vi "Autonomous Independent.vi"   [LabVIEW 2016]
doc: "This VI is called when autonomous begins, and will automatically be terminated when autonomous ends. You can carry out timed or sensor driven robot movement independently without needing to return to the caller."
uses:
  <vilib>/Rock Robotics/WPI/Ultrasonic/WPI_UltrasonicRangeUnits.ctl
  <vilib>/Rock Robotics/WPI/ThirdParty/Sensors/navX/_TypeDefs/FRIC_navX_DeviceNumbersTypeDef.ctl
  <vilib>/Rock Robotics/WPI/Utilities/WPI_GetSetVariantRefNum.vi
  <vilib>/Rock Robotics/Network Tables/NT Read String.vi
  <vilib>/Rock Robotics/Network Tables/NT Write Numeric Array.vi
  Robot Global Data.vi
  <vilib>/Rock Robotics/WPI/RobotDrive/WPI_RobotDriveArcadeDrive_Standard(NoSaturation).vi
  <vilib>/Rock Robotics/WPI/Ultrasonic/WPI_SonarSRF04DigitalRefNum Registry Get.vi
  <vilib>/Rock Robotics/WPI/Ultrasonic/WPI_SonarSRF04DigitalGetRange.vi
panel:
  # "Be sure to right-click and choose Data Operations>>Make Current Value default if you want to save the array values with the VI"
types:
  T1 = typedef "WPI_JoystickDevRef.ctl" = cluster{"Device":T2}
  T2 = typedef "WPI_JoystickDeviceEnum.ctl" = enum16{"USB 0", "USB 1", "USB 2", "USB 3", "USB 4", "USB 5"}
  T3 = typedef "WPI_UltrasonicRangeUnits.ctl" = enum16{"inches", "mm"}
  T4 = typedef "WPI_RobotDriveDevRef.ctl" = cluster{"DevStatus":errorcluster, "Motors[]":T5[], "Square Inputs":bool, "Max Output":dbl}
  T5 = typedef "WPI_MotorControlDeviceRef.ctl" = cluster{"DeviceStatus":errorcluster, "Type":T6, "PWM":cluster{"PWM Channel":T7, "DeadBand":T8}, "CAN":cluster{"Device Number":u8, "SetOutput VI Ref":variant, "GetOutput VI Ref":variant, "Enable VI Ref":variant, "Disable VI Ref":variant, "Data":variant}, "Invert":bool}
  T6 = typedef "WPI_MotorControlType.ctl" = enum16{"PWM", "CAN"}
  T7 = typedef "FPGA_DIOPWMChannel.ctl" = enum8{"PWM 0", "PWM 1", "PWM 2", "PWM 3", "PWM 4", "PWM 5", "PWM 6", "PWM 7", "PWM 8", "PWM 9", "PWM MXP 0", "PWM MXP 1", "PWM MXP 2", "PWM MXP 3", "PWM MXP 4", "PWM MXP 5", "PWM MXP 6", "PWM MXP 7", "PWM MXP 8", "PWM MXP 9", "Invalid"}
  T8 = typedef "WPI_PWMDeadband.ctl" = cluster{"Name":string, "maxPositivePwm":i32, "minPositivePwm":i32, "centerPwm":i32, "maxNegativePwm":i32, "minNegativePwm":i32, "angularRange":u16}
  T9 = cluster{"Type":enum16{"Normal Object", "Color Object"}, "Signature":u16, "X":u16, "Y":u16, "Width":u16, "Height":u16, "Angle":u16}[]
  T10 = cluster{"Type":enum16{"Normal Object", "Color Object"}, "Signature":u16, "X":u16, "Y":u16, "Width":u16, "Height":u16, "Angle":u16}
  T11 = typedef "WPI_UltrasonicDeviceRef.ctl" = cluster{"DevStatus":errorcluster, "Ping Channel":T12, "Echo Channel":T12, "CntIndex":T13}
  T12 = typedef "FPGA_DIOChannel.ctl" = enum8{"DIO 0", "DIO 1", "DIO 2", "DIO 3", "DIO 4", "DIO 5", "DIO 6", "DIO 7", "DIO 8", "DIO 9", "DIO MXP 0", "DIO MXP 1", "DIO MXP 2", "DIO MXP 3", "DIO MXP 4", "DIO MXP 5", "DIO MXP 6", "DIO MXP 7", "DIO MXP 8", "DIO MXP 9", "DIO MXP 10", "DIO MXP 11", "DIO MXP 12", "DIO MXP 13", "DIO MXP 14", "DIO MXP 15", "SPI Port CS1", "SPI Port CS2", "SPI Port CS3", "SPI Port MISO", "SPI Port MOSI", "Invalid"}
  T13 = typedef "FPGA_CounterCtrSystemIndex.ctl" = enum8{"Ctr 0", "Ctr 1", "Ctr 2", "Ctr 3", "Ctr 4", "Ctr 5", "Ctr 6", "Ctr 7", "Invalid"}
  T14 = typedef "FRIC_navX_DeviceNumbersTypeDef.ctl" = enum16{"Dev0", "Dev1", "Dev2", "Dev3"}
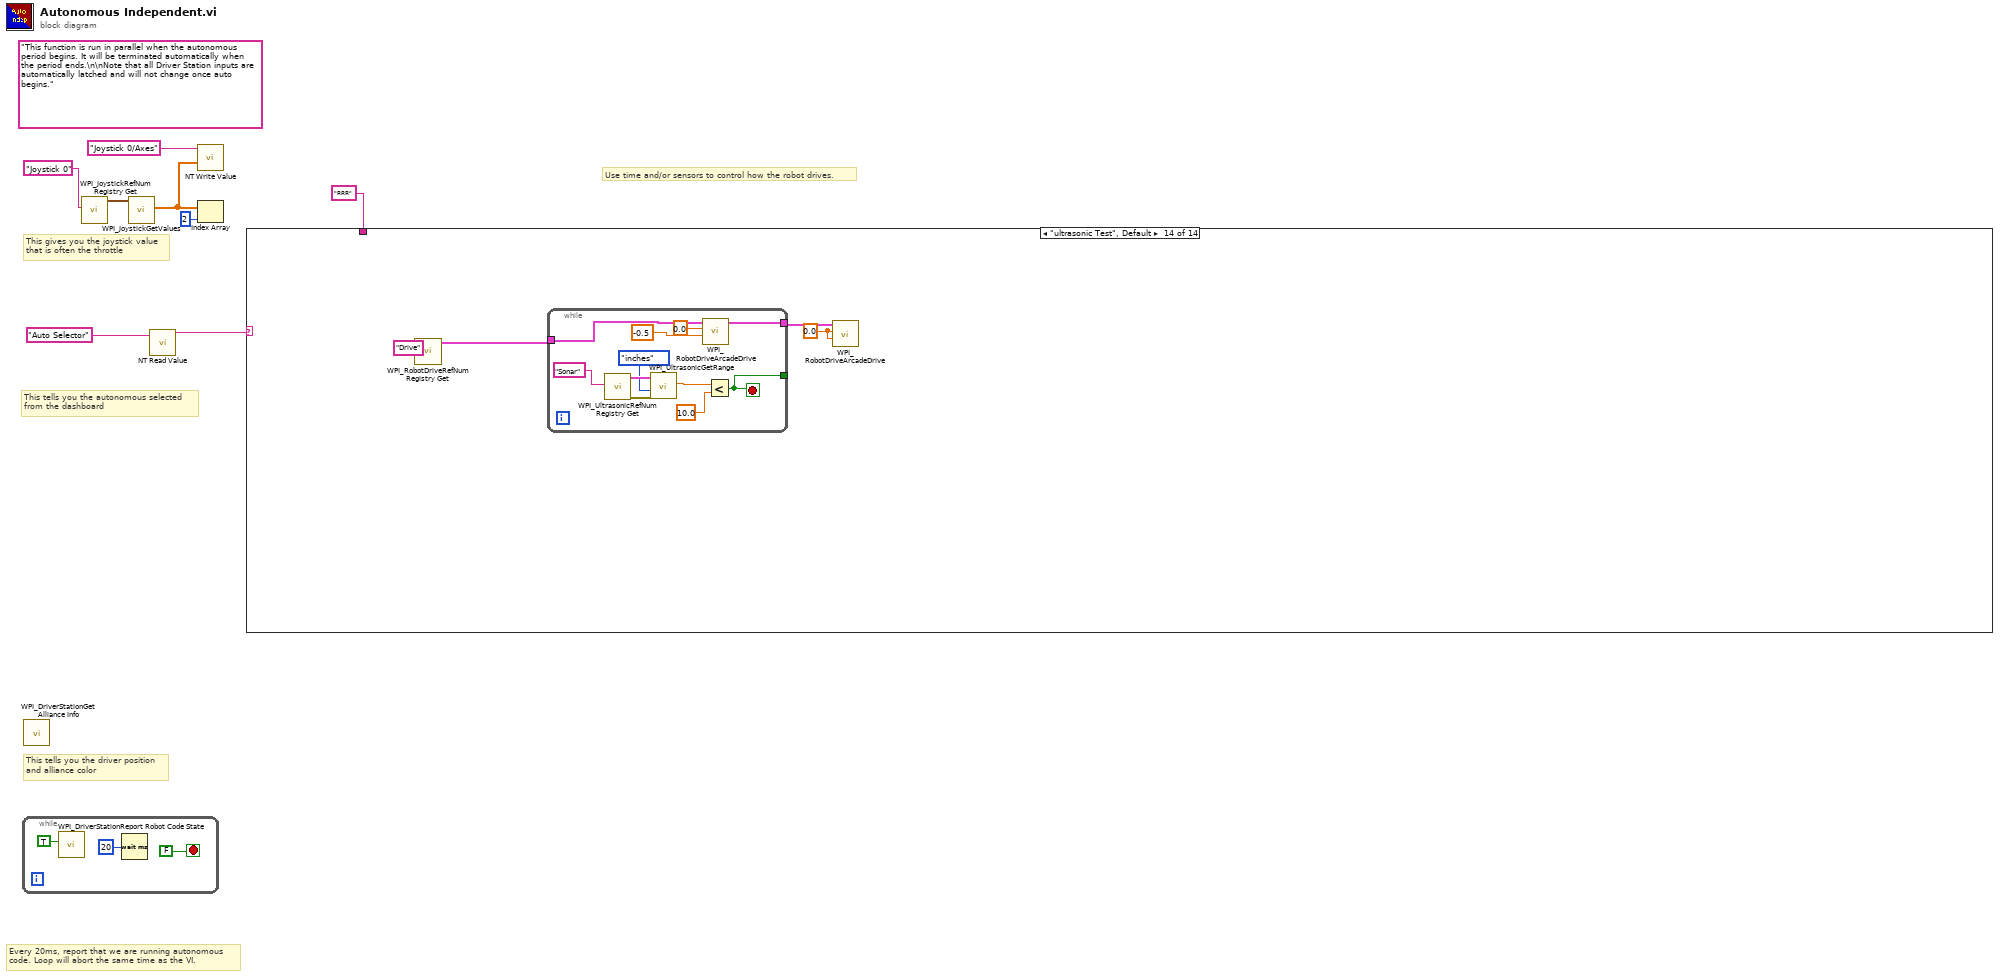
[diagram p0: block diagram]
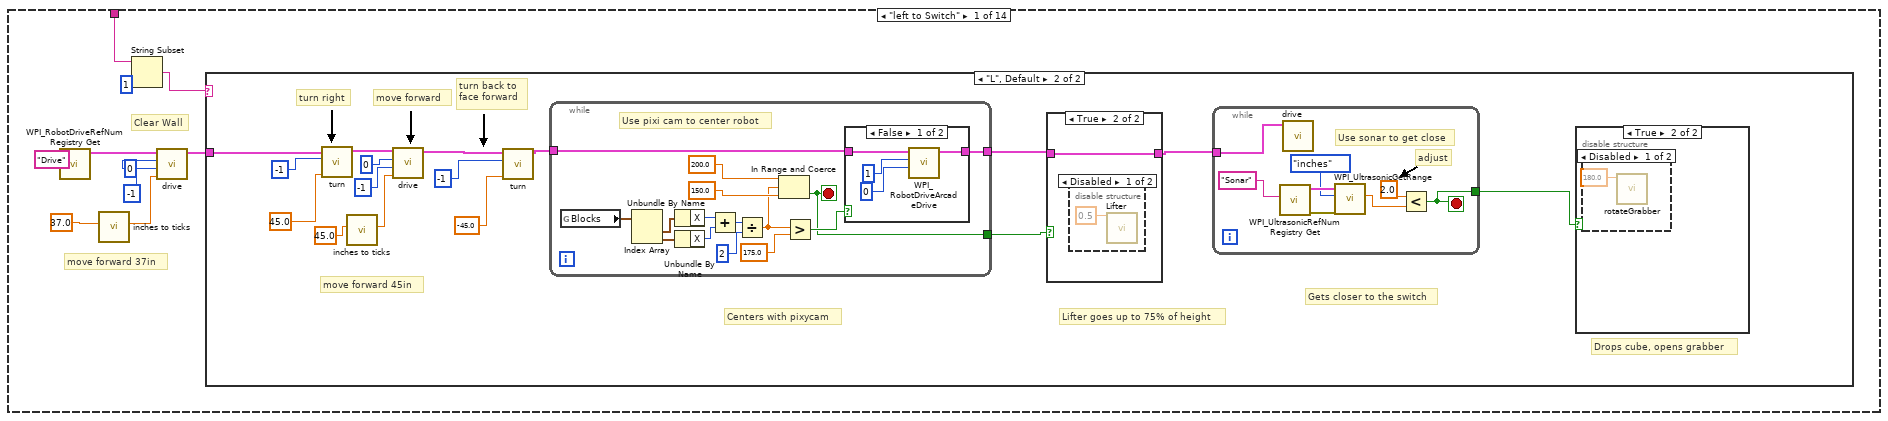
[diagram p2: hidden frame]
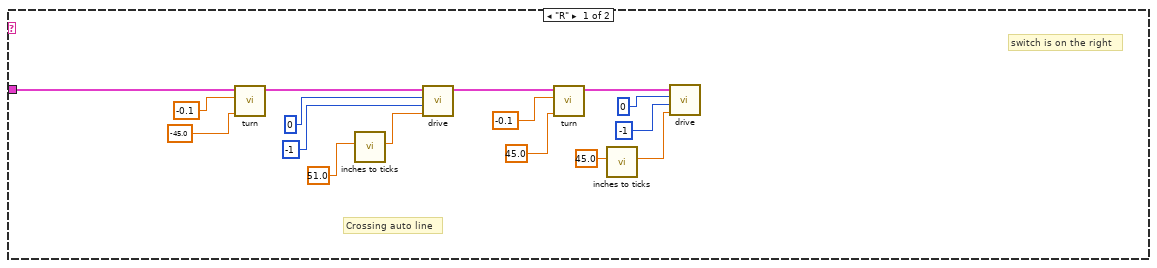
[diagram p3: hidden frame]
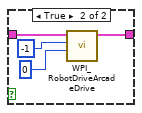
[diagram p8: hidden frame]
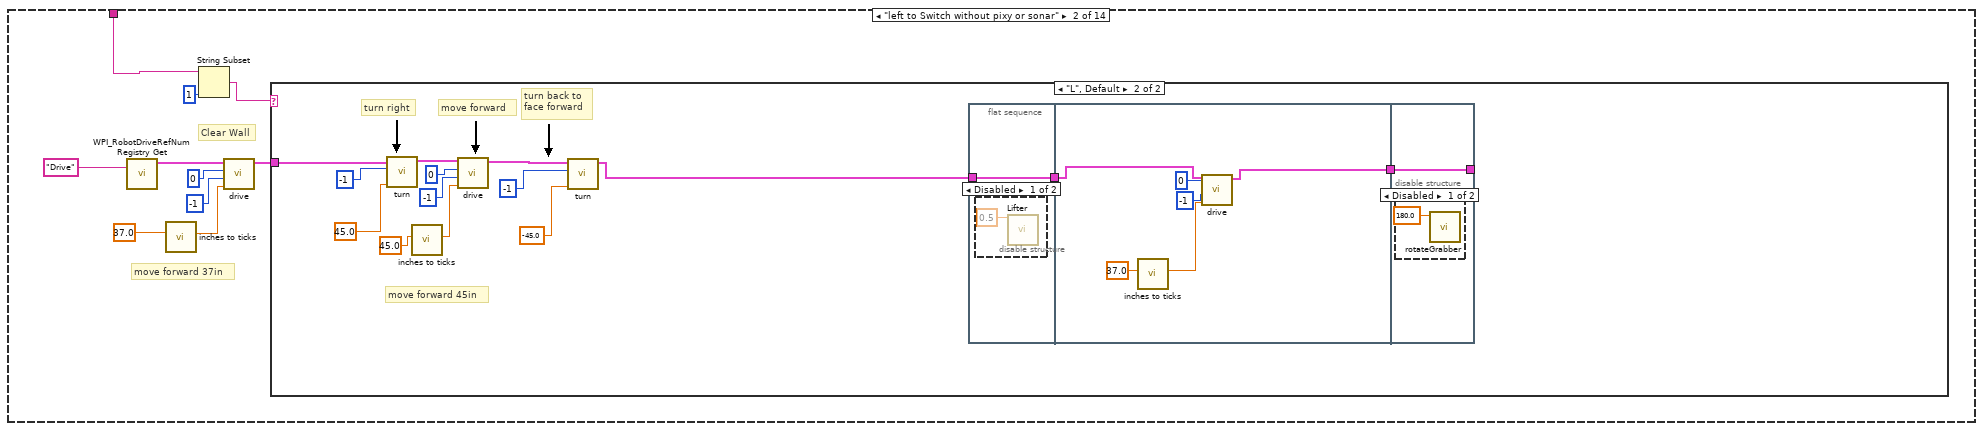
[diagram p9: hidden frame]
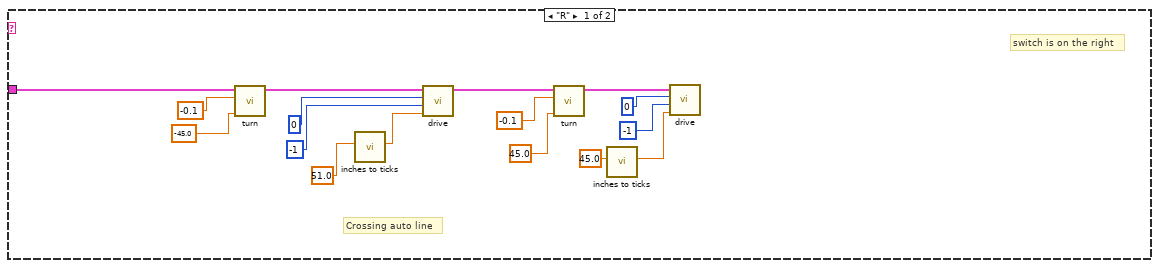
[diagram p10: hidden frame]
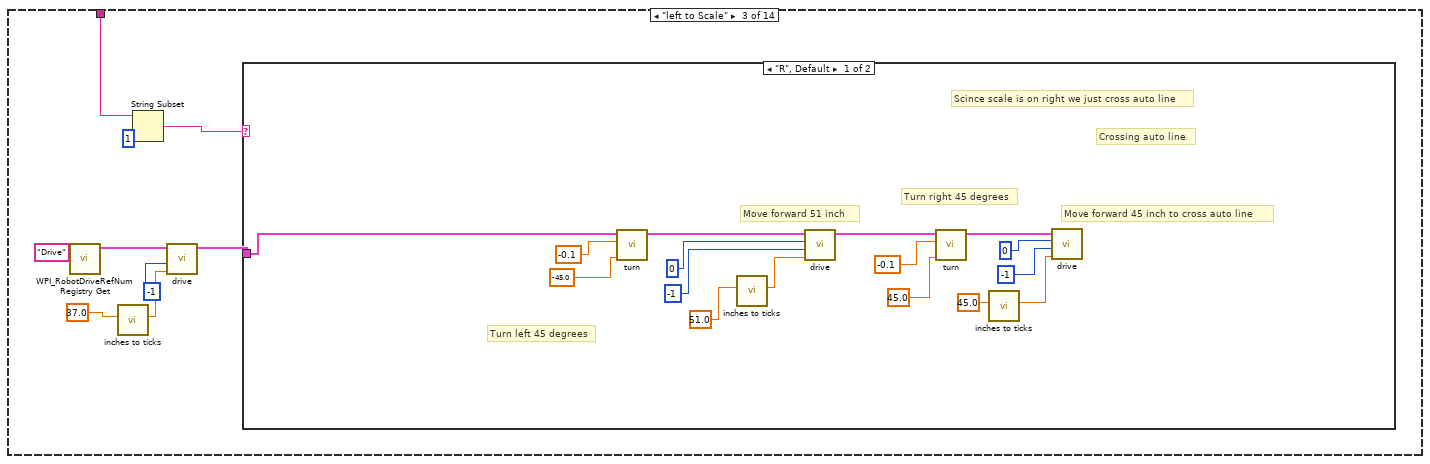
[diagram p13: hidden frame]
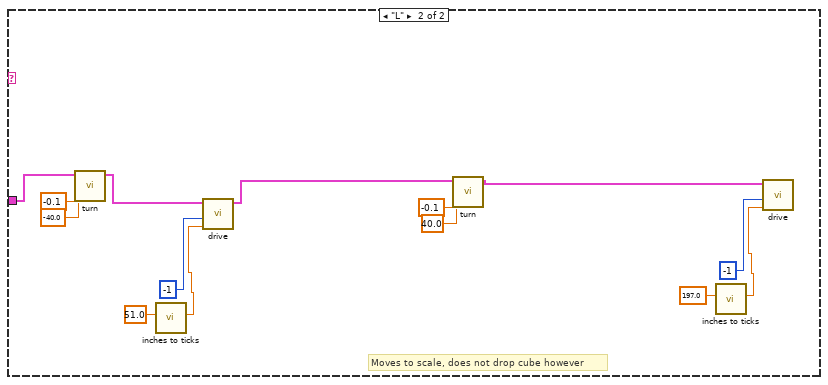
[diagram p14: hidden frame]
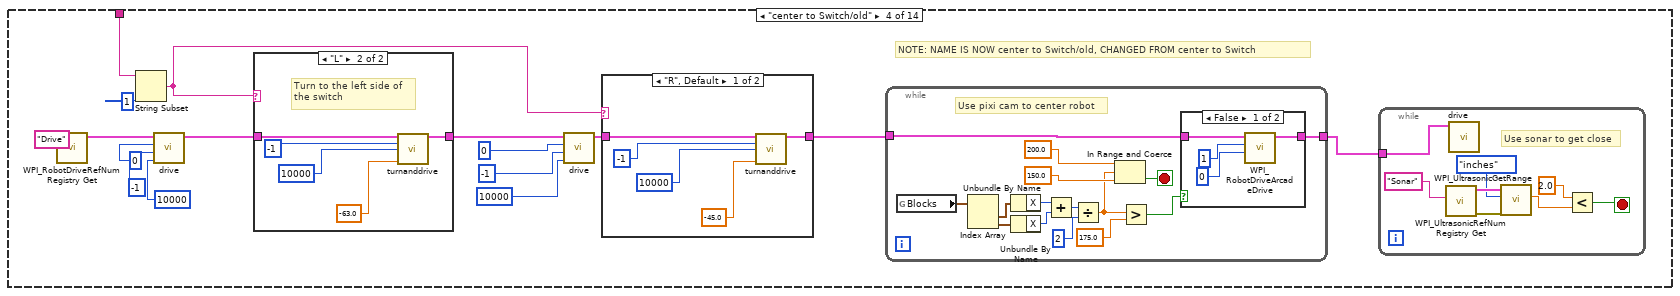
[diagram p15: hidden frame]
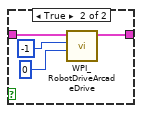
[diagram p16: hidden frame]
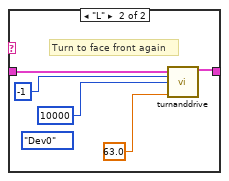
[diagram p17: hidden frame]
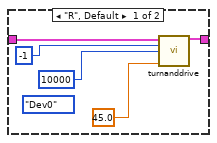
[diagram p18: hidden frame]
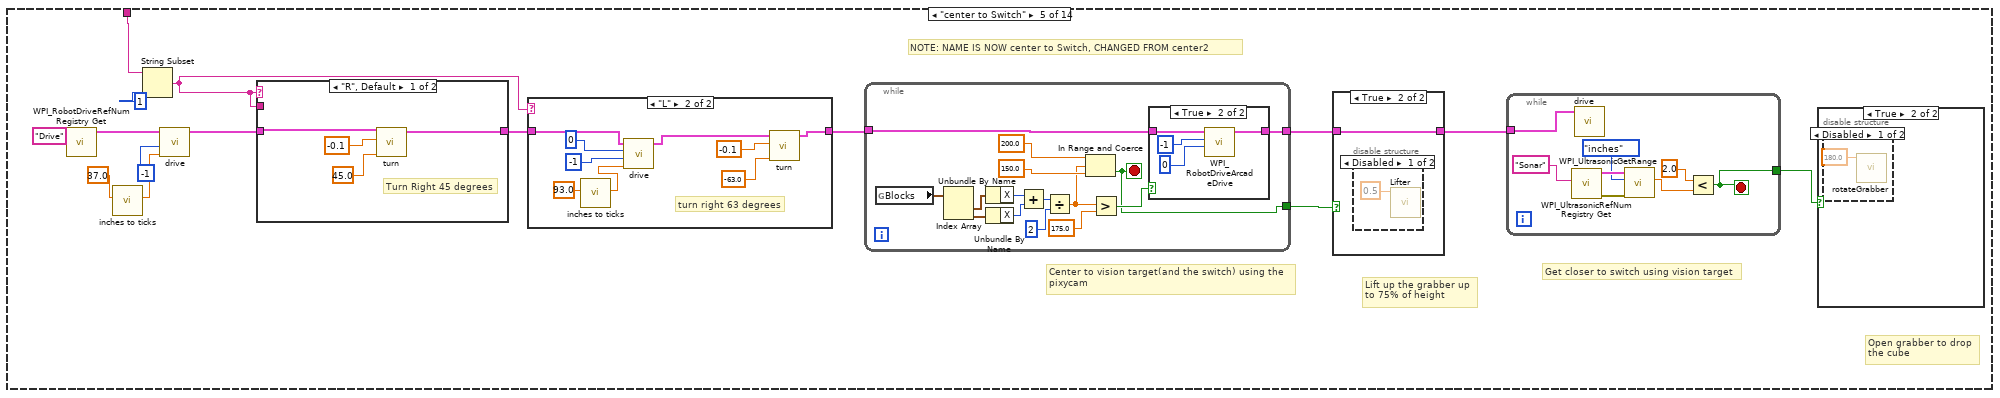
[diagram p19: hidden frame]
diagram:
  (unwired) "This function is run in parallel when the autonomous period begins. It will be terminated automatically when the period ends.\n\nNote that all Driver Station inputs are automatically latched and will not change once auto begins."
  # "This tells you the autonomous selected\nfrom the dashboard"
  # "Every 20ms, report that we are running autonomous\ncode. Loop will abort the same time as the VI."
  # "This gives you the joystick value\nthat is often the throttle"
  # "Use time and/or sensors to control how the robot drives."
  # "This tells you the driver position\nand alliance color"
  n1 = while {
    stop <- FALSE stop-if-true
    n2 = call <vilib>:"WPI_DriverStationReport Robot Code State.vi"("Autonomous"=TRUE) -> ()  [unwired: 10 in, 1 out]
    n3 = Wait (ms)(milliseconds to wait=u32 20) -> ()  [unwired: 1 out]
  }
  n4 = call <vilib>:"WPI_DriverStationGet Alliance Info.vi"() -> ()  [unwired: 12 out]
  n5 = call <vilib>:"WPI_JoystickRefNum Registry Get.vi"("refnum name"="Joystick 0") -> ("JoystickDevRef"=w7:T1)  [unwired: 1 in, 9 out]
  n6 = call <vilib>:"WPI_JoystickGetValues.vi"("JoystickDevRef"=w7) -> ("Axes"=w4:dbl[])  [unwired: 6 in, 4 out]
  n7 = call-poly <vilib>:"NT Read Value.vi"("Name"="Auto Selector") -> ("String"=w2:string)  [unwired: 9 in, 1 out]
  n8 = call-poly <vilib>:"NT Write Value.vi"("Numeric Array"=w4, "Name"="Joystick 0/Axes") -> ()  [unwired: 9 in, 1 out]
  n9 = Index Array(array=w4, index=2) -> ()  [unwired: 1 out]
  n10 = case shown="\"ultrasonic Test\", Default" w2 {
    tunnel: "RRR" ("String") -> [w12 w89 w139 w178 w245 w321 _ _ _ w402 w479 w530 w575 _]
    frame "left to Switch" {
      # "move forward 37in"
      # "Clear Wall"
      n11 = call <vilib>:"WPI_RobotDriveRefNum Registry Get.vi"("refnum name"="Drive") -> ("RobotDriveDevRef"=w20:T4)  [unwired: 9 in, 1 out]
      n12 = call "inches to ticks.vi"("x"=37.0) -> ("x*y"=w14:dbl)  [unwired: 10 in]
      n13 = String Subset(string=w12, length (rest)=1 ("length (rest)")) -> (substring=w15:string)  [unwired: 1 in]
      n14 = call "drive.vi"("distance"=w14, "Y"=-1, "X"=0, "RobotDriveDevRef"=w20) -> ("RobotDriveDevRef dup."=w16:T4)  [unwired: 7 in]
      n15 = case shown="\"L\", Default" w15 {
        tunnel: w16 -> [w22 w53]
        frame "R" {
          # "Crossing auto line"
          # "switch is on the right"
          n16 = call "turn.vi"("Angle"=-45.0, "y"=-0.1, "RobotDriveDevRef"=w22) -> ("RobotDriveDevRef dup."=w31:T4)  [unwired: 8 in]
          n17 = call "inches to ticks.vi"("x"=51.0) -> ("x*y"=w37:dbl)  [unwired: 10 in]
          n18 = call "drive.vi"("distance"=w37, "Y"=-1, "X"=0, "RobotDriveDevRef"=w31) -> ("RobotDriveDevRef dup."=w29:T4)  [unwired: 7 in]
          n19 = call "turn.vi"("Angle"=45.0, "y"=-0.1, "RobotDriveDevRef"=w29) -> ("RobotDriveDevRef dup."=w27:T4)  [unwired: 8 in]
          n20 = call "inches to ticks.vi"("x"=45.0) -> ("x*y"=w26:dbl)  [unwired: 10 in]
          n21 = call "drive.vi"("distance"=w26, "Y"=-1, "X"=0, "RobotDriveDevRef"=w27) -> ()  [unwired: 7 in, 1 out]
        }
        frame "L", Default {
          # "Drops cube, opens grabber"
          # "Gets closer to the switch"
          # "Lifter goes up to 75% of height"
          # "Centers with pixycam"
          # "move forward 45in"
          # "turn back to \nface forward"
          # "move forward"
          # "turn right"
          n22 = call "turn.vi"("Angle"=45.0, "y"=-1, "RobotDriveDevRef"=w53) -> ("RobotDriveDevRef dup."=w50:T4)  [unwired: 8 in]
          n23 = call "inches to ticks.vi"("x"=45.0) -> ("x*y"=w43:dbl)  [unwired: 10 in]
          n24 = call "drive.vi"("distance"=w43, "Y"=-1, "X"=0, "RobotDriveDevRef"=w50) -> ("RobotDriveDevRef dup."=w48:T4)  [unwired: 7 in]
          n25 = call "turn.vi"("Angle"=-45.0, "y"=-1, "RobotDriveDevRef"=w48) -> ("RobotDriveDevRef dup."=w45:T4)  [unwired: 8 in]
          n26 = while {
            tunnel: w45 -> [w67]
            tunnel: [w68] -> w41
            tunnel: [w66] -> w39
            stop <- w66 stop-if-true
            # "Use pixi cam to center robot"
            n27 = global read "Robot Global Data.vi" "Blocks"() -> (w80:T9)
            n28 = Index Array(array=w80) -> (element #1=w79:T10, element #2=w78:T10)  [unwired: 2 in]
            n29 = Unbundle By Name(w79) -> ("X"=w77:u16)
            n30 = Unbundle By Name(w78) -> ("X"=w76:u16)
            n31 = Add(x=w77, y=w76) -> (x+y=w75:u16)
            n32 = Divide(x=w75, y=u16 2) -> (x/y=w73:dbl)
            n33 = In Range and Coerce(upper limit=200.0, x=w73, lower limit=150.0) -> (In Range?=w66:bool)  [unwired: 1 out]
            n34 = Greater?(x=w73, y=175.0) -> (0:w71:bool)
            n35 = case shown="False" w71 {
              tunnel: w67 -> [w84 w86]
              tunnel: [w81 w85] -> w68
              frame False {
                n36 = call-poly <vilib>:"WPI_RobotDriveArcadeDrive.vi"("Y axis value"=0, "X axis value"=1, "RobotDriveDevRef"=w84) -> ("RobotDriveDevRef"=w81:T4)  [unwired: 6 in, 2 out]
              }
              frame True {
                n37 = call-poly <vilib>:"WPI_RobotDriveArcadeDrive.vi"("Y axis value"=0, "X axis value"=-1, "RobotDriveDevRef"=w86) -> ("RobotDriveDevRef"=w85:T4)  [unwired: 6 in, 2 out]
              }
            }
          }
          n38 = case shown="True" w39 {
            tunnel: [w55 w56] -> w40
            tunnel: w41 -> [w55 w56]
            frame False {
            }
            frame True {
              n39 = disable-structure shown="Disabled" {
                frame Disabled {
                  n40 = call "Lifter.vi"("Position from -1 to 1"=0.5) -> ()  [unwired: 11 in]
                }
                frame Enabled {
                }
              }
            }
          }
          n41 = while {
            tunnel: w40 -> [w65]
            tunnel: [w58] -> w38
            stop <- w58 stop-if-true
            # "adjust"
            # "Use sonar to get close"
            n42 = call-poly <vilib>:"WPI_UltrasonicRefNum Registry Get.vi"("refnum name"="Sonar") -> ("error out"=w63:errorcluster, "SonarSRF04DevRef"=w64:T11)  [unwired: 9 in]
            n43 = call "drive.vi"("RobotDriveDevRef"=w65) -> ()  [unwired: 10 in, 1 out]
            n44 = call-poly <vilib>:"WPI_UltrasonicGetRange.vi"("error in (no error)"=w63, "ping time (s)"=WPI_UltrasonicRangeUnits."inches" ("Range Units"), "SonarSRF04DevRef"=w64) -> ("Distance"=w61:dbl)  [unwired: 6 in, 2 out]
            n45 = Less?(x=2.0, y=w61) -> (x < y?=w58:bool)
          }
          n46 = case shown="True" w38 {
            frame False {
            }
            frame True {
              n47 = disable-structure shown="Disabled" {
                frame Disabled {
                  n48 = call "rotateGrabber.vi"("Position from 90 to 180"=180.0) -> ()  [unwired: 11 in]
                }
                frame Enabled {
                }
              }
            }
          }
        }
      }
    }
    frame "left to Switch without pixy or sonar" {
      # "move forward 37in"
      # "Clear Wall"
      n49 = call <vilib>:"WPI_RobotDriveRefNum Registry Get.vi"("refnum name"="Drive") -> ("RobotDriveDevRef"=w95:T4)  [unwired: 9 in, 1 out]
      n50 = call "inches to ticks.vi"("x"=37.0) -> ("x*y"=w98:dbl)  [unwired: 10 in]
      n51 = String Subset(string=w89, length (rest)=1 ("length (rest)")) -> (substring=w97:string)  [unwired: 1 in]
      n52 = call "drive.vi"("distance"=w98, "Y"=-1, "X"=0, "RobotDriveDevRef"=w95) -> ("RobotDriveDevRef dup."=w96:T4)  [unwired: 7 in]
      n53 = case shown="\"L\", Default" w97 {
        tunnel: w96 -> [w99 w128]
        frame "R" {
          # "Crossing auto line"
          # "switch is on the right"
          n54 = call "turn.vi"("Angle"=-45.0, "y"=-0.1, "RobotDriveDevRef"=w99) -> ("RobotDriveDevRef dup."=w108:T4)  [unwired: 8 in]
          n55 = call "inches to ticks.vi"("x"=51.0) -> ("x*y"=w114:dbl)  [unwired: 10 in]
          n56 = call "drive.vi"("distance"=w114, "Y"=-1, "X"=0, "RobotDriveDevRef"=w108) -> ("RobotDriveDevRef dup."=w106:T4)  [unwired: 7 in]
          n57 = call "turn.vi"("Angle"=45.0, "y"=-0.1, "RobotDriveDevRef"=w106) -> ("RobotDriveDevRef dup."=w104:T4)  [unwired: 8 in]
          n58 = call "inches to ticks.vi"("x"=45.0) -> ("x*y"=w103:dbl)  [unwired: 10 in]
          n59 = call "drive.vi"("distance"=w103, "Y"=-1, "X"=0, "RobotDriveDevRef"=w104) -> ()  [unwired: 7 in, 1 out]
        }
        frame "L", Default {
          # "move forward 45in"
          # "turn back to \nface forward"
          # "move forward"
          # "turn right"
          n60 = call "turn.vi"("Angle"=45.0, "y"=-1, "RobotDriveDevRef"=w128) -> ("RobotDriveDevRef dup."=w125:T4)  [unwired: 8 in]
          n61 = call "inches to ticks.vi"("x"=45.0) -> ("x*y"=w119:dbl)  [unwired: 10 in]
          n62 = call "drive.vi"("distance"=w119, "Y"=-1, "X"=0, "RobotDriveDevRef"=w125) -> ("RobotDriveDevRef dup."=w123:T4)  [unwired: 7 in]
          n63 = call "turn.vi"("Angle"=-45.0, "y"=-1, "RobotDriveDevRef"=w123) -> ("RobotDriveDevRef dup."=w116:T4)  [unwired: 8 in]
          n64 = flat-sequence {
            tunnel: [w129] -> w117
            tunnel: w116 -> [w129]
            tunnel: w117 -> [w132]
            tunnel: [w131] -> w115
            tunnel: w115 -> [w137]
            tunnel: [w137] -> _
            frame #0 {
              n65 = disable-structure shown="Disabled" {
                frame Disabled {
                  n66 = call "Lifter.vi"("Position from -1 to 1"=0.5) -> ()  [unwired: 11 in]
                }
                frame Enabled {
                }
              }
            }
            frame #1 {
              n67 = call "inches to ticks.vi"("x"=37.0) -> ("x*y"=w136:dbl)  [unwired: 10 in]
              n68 = call "drive.vi"("distance"=w136, "Y"=-1, "X"=0, "RobotDriveDevRef"=w132) -> ("RobotDriveDevRef dup."=w131:T4)  [unwired: 7 in]
            }
            frame #2 {
              n69 = disable-structure shown="Disabled" {
                frame Disabled {
                  n70 = call "rotateGrabber.vi"("Position from 90 to 180"=180.0) -> ()  [unwired: 11 in]
                }
                frame Enabled {
                }
              }
            }
          }
        }
      }
    }
    frame "left to Scale" {
      n71 = call <vilib>:"WPI_RobotDriveRefNum Registry Get.vi"("refnum name"="Drive") -> ("RobotDriveDevRef"=w144:T4)  [unwired: 9 in, 1 out]
      n72 = call "inches to ticks.vi"("x"=37.0) -> ("x*y"=w145:dbl)  [unwired: 10 in]
      n73 = String Subset(string=w139, length (rest)=1 ("length (rest)")) -> (substring=w146:string)  [unwired: 1 in]
      n74 = call "drive.vi"("distance"=w145, "Y"=-1, "RobotDriveDevRef"=w144) -> ("RobotDriveDevRef dup."=w140:T4)  [unwired: 8 in]
      n75 = case shown="\"R\", Default" w146 {
        tunnel: w140 -> [w148 w177]
        frame "R", Default {
          # "Move forward 45 inch to cross auto line"
          # "Turn right 45 degrees"
          # "Move forward 51 inch"
          # "Turn left 45 degrees"
          # "Scince scale is on right we just cross auto line"
          # "Crossing auto line"
          n76 = call "turn.vi"("Angle"=-45.0, "y"=-0.1, "RobotDriveDevRef"=w148) -> ("RobotDriveDevRef dup."=w157:T4)  [unwired: 8 in]
          n77 = call "inches to ticks.vi"("x"=51.0) -> ("x*y"=w163:dbl)  [unwired: 10 in]
          n78 = call "drive.vi"("distance"=w163, "Y"=-1, "X"=0, "RobotDriveDevRef"=w157) -> ("RobotDriveDevRef dup."=w155:T4)  [unwired: 7 in]
          n79 = call "turn.vi"("Angle"=45.0, "y"=-0.1, "RobotDriveDevRef"=w155) -> ("RobotDriveDevRef dup."=w153:T4)  [unwired: 8 in]
          n80 = call "inches to ticks.vi"("x"=45.0) -> ("x*y"=w152:dbl)  [unwired: 10 in]
          n81 = call "drive.vi"("distance"=w152, "Y"=-1, "X"=0, "RobotDriveDevRef"=w153) -> ()  [unwired: 7 in, 1 out]
        }
        frame "L" {
          # "Moves to scale, does not drop cube however"
          n82 = call "turn.vi"("Angle"=-40.0, "y"=-0.1, "RobotDriveDevRef"=w177) -> ("RobotDriveDevRef dup."=w174:T4)  [unwired: 8 in]
          n83 = call "inches to ticks.vi"("x"=51.0) -> ("x*y"=w171:dbl)  [unwired: 10 in]
          n84 = call "drive.vi"("distance"=w171, "Y"=-1, "RobotDriveDevRef"=w174) -> ("RobotDriveDevRef dup."=w168:T4)  [unwired: 8 in]
          n85 = call "turn.vi"("Angle"=40.0, "y"=-0.1, "RobotDriveDevRef"=w168) -> ("RobotDriveDevRef dup."=w164:T4)  [unwired: 8 in]
          n86 = call "inches to ticks.vi"("x"=197.0) -> ("x*y"=w165:dbl)  [unwired: 10 in]
          n87 = call "drive.vi"("distance"=w165, "Y"=-1, "RobotDriveDevRef"=w164) -> ()  [unwired: 8 in, 1 out]
        }
      }
    }
    frame "center to Switch/old" {
      # "NOTE: NAME IS NOW center to Switch/old, CHANGED FROM center to Switch"
      n88 = call <vilib>:"WPI_RobotDriveRefNum Registry Get.vi"("refnum name"="Drive") -> ("RobotDriveDevRef"=w188:T4)  [unwired: 9 in, 1 out]
      n89 = String Subset(string=w178, length (rest)=1 ("length (rest)")) -> (substring=w190:string)  [unwired: 1 in]
      n90 = call "drive.vi"("distance"=10000, "Y"=-1, "X"=0, "RobotDriveDevRef"=w188) -> ("RobotDriveDevRef dup."=w189:T4)  [unwired: 7 in]
      n91 = case shown="\"L\"" w190 {
        tunnel: w189 -> [w237 w244]
        tunnel: [w236 w243] -> w185
        frame "R", Default {
          (unwired) FRIC_navX_DeviceNumbersTypeDef."Dev0" ("Device Number")
          n92 = call "turnanddrive.vi"("RobotDriveDevRef"=w237, "y"=-1, "distance"=10000, "Angle"=45.0 ("Angel")) -> ("RobotDriveDevRef dup."=w236:T4)  [unwired: 11 in]
        }
        frame "L" {
          # "Turn to the left side of \nthe switch"
          n93 = call "turnanddrive.vi"("RobotDriveDevRef"=w244, "y"=-1, "distance"=10000, "Angle"=-63.0 ("Angel")) -> ("RobotDriveDevRef dup."=w243:T4)  [unwired: 11 in]
        }
      }
      n94 = call "drive.vi"("distance"=10000, "Y"=-1, "X"=0, "RobotDriveDevRef"=w185) -> ("RobotDriveDevRef dup."=w184:T4)  [unwired: 7 in]
      n95 = case shown="\"R\", Default" w190 {
        tunnel: w184 -> [w226 w232]
        tunnel: [w225 w231] -> w191
        frame "R", Default {
          n96 = call "turnanddrive.vi"("RobotDriveDevRef"=w226, "y"=-1, "distance"=10000, "Angle"=-45.0 ("Angel")) -> ("RobotDriveDevRef dup."=w225:T4)  [unwired: 11 in]
        }
        frame "L" {
          (unwired) FRIC_navX_DeviceNumbersTypeDef."Dev0" ("Device Number")
          # "Turn to face front again"
          n97 = call "turnanddrive.vi"("RobotDriveDevRef"=w232, "y"=-1, "distance"=10000, "Angle"=63.0 ("Angel")) -> ("RobotDriveDevRef dup."=w231:T4)  [unwired: 11 in]
        }
      }
      n98 = while {
        tunnel: w191 -> [w202]
        tunnel: [w203] -> w179
        stop <- w209 stop-if-true
        # "Use pixi cam to center robot"
        n99 = global read "Robot Global Data.vi" "Blocks"() -> (w216:T9)
        n100 = Index Array(array=w216) -> (element #1=w215:T10, element #2=w214:T10)  [unwired: 2 in]
        n101 = Unbundle By Name(w215) -> ("X"=w213:u16)
        n102 = Unbundle By Name(w214) -> ("X"=w212:u16)
        n103 = Add(x=w213, y=w212) -> (x+y=w211:u16)
        n104 = Divide(x=w211, y=u16 2) -> (x/y=w208:dbl)
        n105 = In Range and Coerce(upper limit=200.0, x=w208, lower limit=150.0) -> (In Range?=w209:bool)  [unwired: 1 out]
        n106 = Greater?(x=w208, y=175.0) -> (0:w206:bool)
        n107 = case shown="False" w206 {
          tunnel: w202 -> [w220 w222]
          tunnel: [w217 w221] -> w203
          frame False {
            n108 = call-poly <vilib>:"WPI_RobotDriveArcadeDrive.vi"("Y axis value"=0, "X axis value"=1, "RobotDriveDevRef"=w220) -> ("RobotDriveDevRef"=w217:T4)  [unwired: 6 in, 2 out]
          }
          frame True {
            n109 = call-poly <vilib>:"WPI_RobotDriveArcadeDrive.vi"("Y axis value"=0, "X axis value"=-1, "RobotDriveDevRef"=w222) -> ("RobotDriveDevRef"=w221:T4)  [unwired: 6 in, 2 out]
          }
        }
      }
      n110 = while {
        tunnel: w179 -> [w201]
        stop <- w195 stop-if-true
        # "Use sonar to get close"
        n111 = call-poly <vilib>:"WPI_UltrasonicRefNum Registry Get.vi"("refnum name"="Sonar") -> ("error out"=w199:errorcluster, "SonarSRF04DevRef"=w200:T11)  [unwired: 9 in]
        n112 = call "drive.vi"("RobotDriveDevRef"=w201) -> ()  [unwired: 10 in, 1 out]
        n113 = call-poly <vilib>:"WPI_UltrasonicGetRange.vi"("error in (no error)"=w199, "ping time (s)"=WPI_UltrasonicRangeUnits."inches" ("Range Units"), "SonarSRF04DevRef"=w200) -> ("Distance"=w197:dbl)  [unwired: 6 in, 2 out]
        n114 = Less?(x=2.0, y=w197) -> (x < y?=w195:bool)
      }
    }
    frame "center to Switch" {
      # "NOTE: NAME IS NOW center to Switch, CHANGED FROM center2"
      # "Open grabber to drop\nthe cube"
      # "Get closer to switch using vision target"
      # "Lift up the grabber up\nto 75% of height"
      # "Center to vision target(and the switch) using the\npixycam"
      n115 = call <vilib>:"WPI_RobotDriveRefNum Registry Get.vi"("refnum name"="Drive") -> ("RobotDriveDevRef"=w255:T4)  [unwired: 9 in, 1 out]
      n116 = call "inches to ticks.vi"("x"=37.0) -> ("x*y"=w252:dbl)  [unwired: 10 in]
      n117 = String Subset(string=w245, length (rest)=1 ("length (rest)")) -> (substring=w253:string)  [unwired: 1 in]
      n118 = call "drive.vi"("distance"=w252, "Y"=-1, "RobotDriveDevRef"=w255) -> ("RobotDriveDevRef dup."=w256:T4)  [unwired: 8 in]
      n119 = case shown="\"R\", Default" w253 {
        tunnel: w256 -> [w313 w319]
        tunnel: [w314 w320] -> w250
        tunnel: w253 -> [_ _]
        frame "R", Default {
          # "Turn Right 45 degrees"
          n120 = call "turn.vi"("Angle"=45.0, "y"=-0.1, "RobotDriveDevRef"=w313) -> ("RobotDriveDevRef dup."=w314:T4)  [unwired: 8 in]
        }
        frame "L" {
          # "turn left 63 degrees"
          n121 = call "turn.vi"("Angle"=-63.0, "y"=-0.1, "RobotDriveDevRef"=w319) -> ("RobotDriveDevRef dup."=w320:T4)  [unwired: 8 in]
        }
      }
      n122 = case shown="\"L\"" w253 {
        tunnel: w250 -> [w298 w305]
        tunnel: [w301 w310] -> w257
        frame "R", Default {
          # "Turn left 45 degrees"
          n123 = call "inches to ticks.vi"("x"=41.0) -> ("x*y"=w295:dbl)  [unwired: 10 in]
          n124 = call "drive.vi"("distance"=w295, "Y"=-1, "X"=0, "RobotDriveDevRef"=w298) -> ("RobotDriveDevRef dup."=w297:T4)  [unwired: 7 in]
          n125 = call "turn.vi"("Angle"=-45.0, "y"=-0.1, "RobotDriveDevRef"=w297) -> ("RobotDriveDevRef dup."=w301:T4)  [unwired: 8 in]
        }
        frame "L" {
          # "turn right 63 degrees"
          n126 = call "inches to ticks.vi"("x"=93.0) -> ("x*y"=w307:dbl)  [unwired: 10 in]
          n127 = call "drive.vi"("distance"=w307, "Y"=-1, "X"=0, "RobotDriveDevRef"=w305) -> ("RobotDriveDevRef dup."=w304:T4)  [unwired: 7 in]
          n128 = call "turn.vi"("Angle"=-63.0, "y"=-0.1, "RobotDriveDevRef"=w304) -> ("RobotDriveDevRef dup."=w310:T4)  [unwired: 8 in]
        }
      }
      n129 = while {
        tunnel: w257 -> [w274]
        tunnel: [w275] -> w246
        tunnel: [w272] -> w249
        stop <- w272 stop-if-true
        n130 = global read "Robot Global Data.vi" "Blocks"() -> (w286:T9)
        n131 = Index Array(array=w286) -> (element #1=w285:T10, element #2=w284:T10)  [unwired: 2 in]
        n132 = Unbundle By Name(w285) -> ("X"=w283:u16)
        n133 = Unbundle By Name(w284) -> ("X"=w282:u16)
        n134 = Add(x=w283, y=w282) -> (x+y=w281:u16)
        n135 = Divide(x=w281, y=u16 2) -> (x/y=w279:dbl)
        n136 = In Range and Coerce(upper limit=200.0, x=w279, lower limit=150.0) -> (In Range?=w272:bool)  [unwired: 1 out]
        n137 = Greater?(x=w279, y=175.0) -> (0:w273:bool)
        n138 = case shown="True" w273 {
          tunnel: w274 -> [w290 w292]
          tunnel: [w287 w291] -> w275
          frame False {
            n139 = call-poly <vilib>:"WPI_RobotDriveArcadeDrive.vi"("Y axis value"=0, "X axis value"=1, "RobotDriveDevRef"=w290) -> ("RobotDriveDevRef"=w287:T4)  [unwired: 6 in, 2 out]
          }
          frame True {
            n140 = call-poly <vilib>:"WPI_RobotDriveArcadeDrive.vi"("Y axis value"=0, "X axis value"=-1, "RobotDriveDevRef"=w292) -> ("RobotDriveDevRef"=w291:T4)  [unwired: 6 in, 2 out]
          }
        }
      }
      n141 = case shown="True" w249 {
        tunnel: [w261 w262] -> w247
        tunnel: w246 -> [w261 w262]
        frame False {
        }
        frame True {
          n142 = disable-structure shown="Disabled" {
            frame Disabled {
              n143 = call "Lifter.vi"("Position from -1 to 1"=0.5) -> ()  [unwired: 11 in]
            }
            frame Enabled {
            }
          }
        }
      }
      n144 = while {
        tunnel: w247 -> [w271]
        tunnel: [w264] -> w248
        stop <- w264 stop-if-true
        n145 = call-poly <vilib>:"WPI_UltrasonicRefNum Registry Get.vi"("refnum name"="Sonar") -> ("error out"=w269:errorcluster, "SonarSRF04DevRef"=w270:T11)  [unwired: 9 in]
        n146 = call "drive.vi"("RobotDriveDevRef"=w271) -> ()  [unwired: 10 in, 1 out]
        n147 = call-poly <vilib>:"WPI_UltrasonicGetRange.vi"("error in (no error)"=w269, "ping time (s)"=WPI_UltrasonicRangeUnits."inches" ("Range Units"), "SonarSRF04DevRef"=w270) -> ("Distance"=w267:dbl)  [unwired: 6 in, 2 out]
        n148 = Less?(x=2.0, y=w267) -> (x < y?=w264:bool)
      }
      n149 = case shown="True" w248 {
        frame False {
        }
        frame True {
          n150 = disable-structure shown="Disabled" {
            frame Disabled {
              n151 = call "rotateGrabber.vi"("Position from 90 to 180"=180.0) -> ()  [unwired: 11 in]
            }
            frame Enabled {
            }
          }
        }
      }
    }
    frame "center to Switch without pixy or sonar" {
      n152 = call <vilib>:"WPI_RobotDriveRefNum Registry Get.vi"("refnum name"="Drive") -> ("RobotDriveDevRef"=w330:T4)  [unwired: 9 in, 1 out]
      n153 = call "inches to ticks.vi"("x"=37.0) -> ("x*y"=w332:dbl)  [unwired: 10 in]
      n154 = String Subset(string=w321, length (rest)=1 ("length (rest)")) -> (substring=w331:string)  [unwired: 1 in]
      n155 = call "drive.vi"("distance"=w332, "Y"=-1, "RobotDriveDevRef"=w330) -> ("RobotDriveDevRef dup."=w329:T4)  [unwired: 8 in]
      n156 = case shown="\"L\"" w331 {
        tunnel: w329 -> [w362 w368]
        tunnel: [w363 w369] -> w333
        tunnel: w331 -> [_ _]
        frame "R", Default {
          # "Turn Right 45 degrees"
          n157 = call "turn.vi"("Angle"=45.0, "y"=-0.1, "RobotDriveDevRef"=w362) -> ("RobotDriveDevRef dup."=w363:T4)  [unwired: 8 in]
        }
        frame "L" {
          # "turn left 63 degrees"
          n158 = call "turn.vi"("Angle"=-63.0, "y"=-0.1, "RobotDriveDevRef"=w368) -> ("RobotDriveDevRef dup."=w369:T4)  [unwired: 8 in]
        }
      }
      n159 = case shown="\"R\", Default" w331 {
        tunnel: w333 -> [w347 w354]
        tunnel: [w350 w359] -> w322
        frame "R", Default {
          # "Turn left 45 degrees"
          n160 = call "inches to ticks.vi"("x"=41.0) -> ("x*y"=w344:dbl)  [unwired: 10 in]
          n161 = call "drive.vi"("distance"=w344, "Y"=-1, "X"=0, "RobotDriveDevRef"=w347) -> ("RobotDriveDevRef dup."=w346:T4)  [unwired: 7 in]
          n162 = call "turn.vi"("Angle"=-45.0, "y"=-0.1, "RobotDriveDevRef"=w346) -> ("RobotDriveDevRef dup."=w350:T4)  [unwired: 8 in]
        }
        frame "L" {
          # "turn right 63 degrees"
          n163 = call "inches to ticks.vi"("x"=93.0) -> ("x*y"=w356:dbl)  [unwired: 10 in]
          n164 = call "drive.vi"("distance"=w356, "Y"=-1, "X"=0, "RobotDriveDevRef"=w354) -> ("RobotDriveDevRef dup."=w353:T4)  [unwired: 7 in]
          n165 = call "turn.vi"("Angle"=-63.0, "y"=-0.1, "RobotDriveDevRef"=w353) -> ("RobotDriveDevRef dup."=w359:T4)  [unwired: 8 in]
        }
      }
      n166 = flat-sequence {
        tunnel: [w334] -> w323
        tunnel: w322 -> [w334]
        tunnel: [w337] -> w324
        tunnel: w323 -> [w336]
        tunnel: [w342] -> _
        tunnel: w324 -> [w342]
        frame #0 {
          n167 = disable-structure shown="Disabled" {
            frame Disabled {
              n168 = call "Lifter.vi"("Position from -1 to 1"=0.5) -> ()  [unwired: 11 in]
            }
            frame Enabled {
            }
          }
        }
        frame #1 {
          n169 = call "inches to ticks.vi"("x"=27.0) -> ("x*y"=w341:dbl)  [unwired: 10 in]
          n170 = call "drive.vi"("distance"=w341, "Y"=-1, "X"=0, "RobotDriveDevRef"=w336) -> ("RobotDriveDevRef dup."=w337:T4)  [unwired: 7 in]
        }
        frame #2 {
          n171 = disable-structure shown="Disabled" {
            frame Disabled {
              n172 = call "rotateGrabber.vi"("Position from 90 to 180"=180.0) -> ()  [unwired: 11 in]
            }
            frame Enabled {
            }
          }
        }
      }
    }
    frame "center to Cross Line Left" {
      # "Turn right 63 degrees"
      # "Turn left 63 degrees"
      n173 = call <vilib>:"WPI_RobotDriveRefNum Registry Get.vi"("refnum name"="Drive") -> ("RobotDriveDevRef"=w390:T4)  [unwired: 9 in, 1 out]
      n174 = call "inches to ticks.vi"("x"=37.0) -> ("x*y"=w391:dbl)  [unwired: 10 in]
      n175 = call "drive.vi"("distance"=w391, "Y"=-1, "X"=0, "RobotDriveDevRef"=w390) -> ("RobotDriveDevRef dup."=w376:T4)  [unwired: 7 in]
      n176 = call "turn.vi"("Angle"=-63.0, "y"=-0.1, "RobotDriveDevRef"=w376) -> ("RobotDriveDevRef dup."=w375:T4)  [unwired: 8 in]
      n177 = call "inches to ticks.vi"("x"=149.0) -> ("x*y"=w384:dbl)  [unwired: 10 in]
      n178 = call "drive.vi"("distance"=w384, "Y"=-1, "X"=0, "RobotDriveDevRef"=w375) -> ("RobotDriveDevRef dup."=w385:T4)  [unwired: 7 in]
      n179 = call "turn.vi"("Angle"=-63.0, "y"=-0.1, "RobotDriveDevRef"=w385) -> ("RobotDriveDevRef dup."=w373:T4)  [unwired: 8 in]
      n180 = call "inches to ticks.vi"("x"=37.0) -> ("x*y"=w374:dbl)  [unwired: 10 in]
      n181 = call "drive.vi"("distance"=w374, "Y"=-1, "X"=0, "RobotDriveDevRef"=w373) -> ()  [unwired: 7 in, 1 out]
    }
    frame "turn test" {
      # "Test the turn block"
      n182 = call <vilib>:"WPI_RobotDriveRefNum Registry Get.vi"("refnum name"="Drive") -> ("RobotDriveDevRef"=w394:T4)  [unwired: 9 in, 1 out]
      n183 = call "turn.vi"("Angle"=-45.0, "y"=0, "RobotDriveDevRef"=w394) -> ()  [unwired: 8 in, 1 out]
    }
    frame "drive forward" {
      n184 = call <vilib>:"WPI_RobotDriveRefNum Registry Get.vi"("refnum name"="Drive") -> ("RobotDriveDevRef"=w401:T4)  [unwired: 9 in, 1 out]
      n185 = call "inches to ticks.vi"("x"=24.0) -> ("x*y"=w398:dbl)  [unwired: 10 in]
      n186 = call "drive.vi"("distance"=w398, "Y"=-0.5, "X"=0.0, "RobotDriveDevRef"=w401) -> ()  [unwired: 7 in, 1 out]
    }
    frame "right to Switch" {
      # "If our side of switch is on left, then cross the auto line or attempt to score scale if our side of the scale is on the right."
      n187 = call <vilib>:"WPI_RobotDriveRefNum Registry Get.vi"("refnum name"="Drive") -> ("RobotDriveDevRef"=w410:T4)  [unwired: 9 in, 1 out]
      n188 = String Subset(string=w402, length (rest)=1 ("length (rest)")) -> (substring=w404:string)  [unwired: 1 in]
      n189 = call "inches to ticks.vi"("x"=37.0) -> ("x*y"=w405:dbl)  [unwired: 10 in]
      n190 = call "drive.vi"("distance"=w405, "Y"=-1, "X"=0, "RobotDriveDevRef"=w410) -> ("RobotDriveDevRef dup."=w403:T4)  [unwired: 7 in]
      n191 = case shown="\"R\", Default" w404 {
        tunnel: w403 -> [w422 w443]
        frame "L" {
          # "Move forward 67 inches \nto cross auto line"
          # "Turn left \n30 degrees"
          # "Move forward \n36 in."
          # "Turn Right 30 degrees"
          # "switch is on the left"
          # "since the switch is on the left we just cross the auto line"
          n192 = call "turn.vi"("Angle"=30.0, "y"=-0.1, "RobotDriveDevRef"=w422) -> ("RobotDriveDevRef dup."=w420:T4)  [unwired: 8 in]
          n193 = call "inches to ticks.vi"("x"=36.0) -> ("x*y"=w427:dbl)  [unwired: 10 in]
          n194 = call "drive.vi"("distance"=w427, "Y"=-1, "X"=0, "RobotDriveDevRef"=w420) -> ("RobotDriveDevRef dup."=w418:T4)  [unwired: 7 in]
          n195 = call "turn.vi"("Angle"=-30.0, "y"=-0.1, "RobotDriveDevRef"=w418) -> ("RobotDriveDevRef dup."=w416:T4)  [unwired: 8 in]
          n196 = call "inches to ticks.vi"("x"=67.0) -> ("x*y"=w415:dbl)  [unwired: 10 in]
          n197 = call "drive.vi"("distance"=w415, "Y"=-1, "X"=0, "RobotDriveDevRef"=w416) -> ()  [unwired: 7 in, 1 out]
        }
        frame "R", Default {
          # "Get closer to the switch"
          # "Opens grabber"
          # "Lift grabber to 75% of height"
          n198 = call "inches to ticks.vi"("x"=55.0) -> ("x*y"=w437:dbl)  [unwired: 10 in]
          n199 = call "turn.vi"("Angle"=-45.0, "y"=-0.1, "RobotDriveDevRef"=w443) -> ("RobotDriveDevRef dup."=w440:T4)  [unwired: 8 in]
          n200 = call "drive.vi"("distance"=w437, "Y"=-1, "X"=0, "RobotDriveDevRef"=w440) -> ("RobotDriveDevRef dup."=w433:T4)  [unwired: 7 in]
          n201 = call "turn.vi"("Angle"=45.0, "y"=-0.1, "RobotDriveDevRef"=w433) -> ("RobotDriveDevRef dup."=w432:T4)  [unwired: 8 in]
          n202 = while {
            tunnel: w432 -> [w455]
            tunnel: [w454] -> w431
            tunnel: [w453] -> w430
            stop <- w454 stop-if-true
            # "Use pixy cam to center robot"
            n203 = global read "Robot Global Data.vi" "Blocks"() -> (w460:T9)
            n204 = Index Array(array=w460) -> (element #1=w461:T10, element #2=w462:T10)  [unwired: 2 in]
            n205 = Unbundle By Name(w461) -> ("X"=w463:u16)
            n206 = Unbundle By Name(w462) -> ("X"=w464:u16)
            n207 = Add(x=w463, y=w464) -> (x+y=w465:u16)
            n208 = Divide(x=w465, y=u16 2) -> (x/y=w466:dbl)
            n209 = In Range and Coerce(upper limit=200.0, x=w466, lower limit=150.0) -> (In Range?=w454:bool)  [unwired: 1 out]
            n210 = Greater?(x=w466, y=175.0) -> (0:w467:bool)
            n211 = case shown="True" w467 {
              tunnel: w455 -> [w471 w473]
              tunnel: [w468 w472] -> w453
              frame False {
                n212 = call-poly <vilib>:"WPI_RobotDriveArcadeDrive.vi"("Y axis value"=0, "X axis value"=1, "RobotDriveDevRef"=w471) -> ("RobotDriveDevRef"=w468:T4)  [unwired: 6 in, 2 out]
              }
              frame True {
                n213 = call-poly <vilib>:"WPI_RobotDriveArcadeDrive.vi"("Y axis value"=0, "X axis value"=-1, "RobotDriveDevRef"=w473) -> ("RobotDriveDevRef"=w472:T4)  [unwired: 6 in, 2 out]
              }
            }
          }
          n214 = case shown="True" w431 {
            tunnel: [w476 w477] -> w429
            tunnel: w430 -> [w476 w477]
            frame False {
            }
            frame True {
              n215 = disable-structure shown="Disabled" {
                frame Disabled {
                  n216 = call "Lifter.vi"("Position from -1 to 1"=0.5) -> ()  [unwired: 11 in]
                }
                frame Enabled {
                }
              }
            }
          }
          n217 = while {
            tunnel: w429 -> [w452]
            tunnel: [w445] -> w428
            stop <- w445 stop-if-true
            n218 = call-poly <vilib>:"WPI_UltrasonicRefNum Registry Get.vi"("refnum name"="Sonar") -> ("error out"=w450:errorcluster, "SonarSRF04DevRef"=w451:T11)  [unwired: 9 in]
            n219 = call "drive.vi"("RobotDriveDevRef"=w452) -> ()  [unwired: 10 in, 1 out]
            n220 = call-poly <vilib>:"WPI_UltrasonicGetRange.vi"("error in (no error)"=w450, "ping time (s)"=WPI_UltrasonicRangeUnits."inches" ("Range Units"), "SonarSRF04DevRef"=w451) -> ("Distance"=w448:dbl)  [unwired: 6 in, 2 out]
            n221 = Less?(x=2.0, y=w448) -> (x < y?=w445:bool)
          }
          n222 = case shown="True" w428 {
            frame False {
            }
            frame True {
              n223 = disable-structure shown="Disabled" {
                frame Disabled {
                  n224 = call "rotateGrabber.vi"("Position from 90 to 180"=180.0) -> ()  [unwired: 11 in]
                }
                frame Enabled {
                }
              }
            }
          }
        }
      }
    }
    frame "right to Switch without pixy or sonar" {
      # "If our side of switch is on left, then cross the auto line or attempt to score scale if our side of the scale is on the right."
      n225 = call <vilib>:"WPI_RobotDriveRefNum Registry Get.vi"("refnum name"="Drive") -> ("RobotDriveDevRef"=w485:T4)  [unwired: 9 in, 1 out]
      n226 = String Subset(string=w479, length (rest)=1 ("length (rest)")) -> (substring=w487:string)  [unwired: 1 in]
      n227 = call "inches to ticks.vi"("x"=37.0) -> ("x*y"=w486:dbl)  [unwired: 10 in]
      n228 = call "drive.vi"("distance"=w486, "Y"=-1, "X"=0, "RobotDriveDevRef"=w485) -> ("RobotDriveDevRef dup."=w488:T4)  [unwired: 7 in]
      n229 = case shown="\"R\", Default" w487 {
        tunnel: w488 -> [w499 w505]
        frame "L" {
          # "Move forward 67 inches \nto cross auto line"
          # "Turn left \n30 degrees"
          # "Move forward \n36 in."
          # "Turn Right 30 degrees"
          # "switch is on the left"
          # "since the switch is on the left we just cross the auto line"
          n230 = call "turn.vi"("Angle"=30.0, "y"=-0.1, "RobotDriveDevRef"=w499) -> ("RobotDriveDevRef dup."=w497:T4)  [unwired: 8 in]
          n231 = call "inches to ticks.vi"("x"=36.0) -> ("x*y"=w504:dbl)  [unwired: 10 in]
          n232 = call "drive.vi"("distance"=w504, "Y"=-1, "X"=0, "RobotDriveDevRef"=w497) -> ("RobotDriveDevRef dup."=w495:T4)  [unwired: 7 in]
          n233 = call "turn.vi"("Angle"=-30.0, "y"=-0.1, "RobotDriveDevRef"=w495) -> ("RobotDriveDevRef dup."=w493:T4)  [unwired: 8 in]
          n234 = call "inches to ticks.vi"("x"=67.0) -> ("x*y"=w492:dbl)  [unwired: 10 in]
          n235 = call "drive.vi"("distance"=w492, "Y"=-1, "X"=0, "RobotDriveDevRef"=w493) -> ()  [unwired: 7 in, 1 out]
        }
        frame "R", Default {
          n236 = disable-structure shown="Enabled" {
            disable-tunnel: w505 -> [w517]
            frame Enabled {
              n237 = call "inches to ticks.vi"("x"=55.0) -> ("x*y"=w511:dbl)  [unwired: 10 in]
              n238 = call "turn.vi"("Angle"=-45.0, "y"=-0.1, "RobotDriveDevRef"=w517) -> ("RobotDriveDevRef dup."=w514:T4)  [unwired: 8 in]
              n239 = call "drive.vi"("distance"=w511, "Y"=-1, "X"=0, "RobotDriveDevRef"=w514) -> ("RobotDriveDevRef dup."=w507:T4)  [unwired: 7 in]
              n240 = call "turn.vi"("Angle"=45.0, "y"=-0.1, "RobotDriveDevRef"=w507) -> ("RobotDriveDevRef dup."=w506:T4)  [unwired: 8 in]
              n241 = flat-sequence {
                tunnel: [w520] -> w519
                tunnel: w506 -> [w520]
                tunnel: w519 -> [w524]
                tunnel: [w523] -> w518
                tunnel: [w528] -> _
                tunnel: w518 -> [w528]
                frame #0 {
                  n242 = disable-structure shown="Disabled" {
                    frame Disabled {
                      n243 = call "Lifter.vi"("Position from -1 to 1"=0.5) -> ()  [unwired: 11 in]
                    }
                    frame Enabled {
                    }
                  }
                }
                frame #1 {
                  n244 = call "inches to ticks.vi"("x"=30.0) -> ("x*y"=w522:dbl)  [unwired: 10 in]
                  n245 = call "drive.vi"("distance"=w522, "Y"=-1, "X"=0, "RobotDriveDevRef"=w524) -> ("RobotDriveDevRef dup."=w523:T4)  [unwired: 7 in]
                }
                frame #2 {
                  n246 = disable-structure shown="Disabled" {
                    frame Disabled {
                      n247 = call "rotateGrabber.vi"("Position from 90 to 180"=180.0) -> ()  [unwired: 11 in]
                    }
                    frame Enabled {
                    }
                  }
                }
              }
            }
          }
        }
      }
    }
    frame "right to Scale" {
      n248 = call <vilib>:"WPI_RobotDriveRefNum Registry Get.vi"("refnum name"="Drive") -> ("RobotDriveDevRef"=w539:T4)  [unwired: 9 in, 1 out]
      n249 = call "inches to ticks.vi"("x"=37.0) -> ("x*y"=w533:dbl)  [unwired: 10 in]
      n250 = String Subset(string=w530, offset (0)=1, length (rest)=1 ("length (rest)")) -> (substring=w535:string)
      n251 = call "drive.vi"("distance"=w533, "Y"=-1, "X"=0, "RobotDriveDevRef"=w539) -> ("RobotDriveDevRef dup."=w531:T4)  [unwired: 7 in]
      n252 = case shown="\"R\", Default" w535 {
        tunnel: w531 -> [w541 w563]
        frame "L" {
          (unwired) FRIC_navX_DeviceNumbersTypeDef."Dev2" ("Device Number")
          (unwired) FRIC_navX_DeviceNumbersTypeDef."Dev2" ("Device Number")
          # "Move forward 67 inches \nto cross auto line"
          # "Turn left \n30 degrees"
          # "Move forward \n36 in."
          # "Turn Right 30 degrees"
          n253 = call "turn.vi"("Angle"=30.0, "y"=-0.1, "RobotDriveDevRef"=w541) -> ("RobotDriveDevRef dup."=w550:T4)  [unwired: 8 in]
          n254 = call "inches to ticks.vi"("x"=36.0) -> ("x*y"=w556:dbl)  [unwired: 10 in]
          n255 = call "drive.vi"("distance"=w556, "Y"=-1, "X"=0, "RobotDriveDevRef"=w550) -> ("RobotDriveDevRef dup."=w548:T4)  [unwired: 7 in]
          n256 = call "turn.vi"("Angle"=-30.0, "y"=-0.1, "RobotDriveDevRef"=w548) -> ("RobotDriveDevRef dup."=w546:T4)  [unwired: 8 in]
          n257 = call "inches to ticks.vi"("x"=67.0) -> ("x*y"=w545:dbl)  [unwired: 10 in]
          n258 = call "drive.vi"("distance"=w545, "Y"=-1, "X"=0, "RobotDriveDevRef"=w546) -> ()  [unwired: 7 in, 1 out]
        }
        frame "R", Default {
          (unwired) FRIC_navX_DeviceNumbersTypeDef."Dev1" ("Device Number")
          (unwired) FRIC_navX_DeviceNumbersTypeDef."Dev1" ("Device Number")
          # "Moves up to the scale, does not drop cube however"
          n259 = call "turn.vi"("Angle"=30.0, "y"=-1, "RobotDriveDevRef"=w563) -> ("RobotDriveDevRef dup."=w562:T4)  [unwired: 8 in]
          n260 = call "inches to ticks.vi"("x"=36.0) -> ("x*y"=w567:dbl)  [unwired: 10 in]
          n261 = call "drive.vi"("distance"=w567, "Y"=-1, "X"=0, "RobotDriveDevRef"=w562) -> ("RobotDriveDevRef dup."=w570:T4)  [unwired: 7 in]
          n262 = call "turn.vi"("Angle"=-30.0, "y"=-1, "RobotDriveDevRef"=w570) -> ("RobotDriveDevRef dup."=w559:T4)  [unwired: 8 in]
          n263 = call "inches to ticks.vi"("x"=201.0) -> ("x*y"=w561:dbl)  [unwired: 10 in]
          n264 = call "drive.vi"("distance"=w561, "Y"=-1, "X"=0, "RobotDriveDevRef"=w559) -> ()  [unwired: 7 in, 1 out]
        }
      }
    }
    frame "right Forward" {
      n265 = call <vilib>:"WPI_RobotDriveRefNum Registry Get.vi"("refnum name"="Drive") -> ("RobotDriveDevRef"=w577:T4)  [unwired: 9 in, 1 out]
      n266 = call "inches to ticks.vi"("x"=24.0) -> ("x*y"=w582:dbl)  [unwired: 10 in]
      n267 = call "drive.vi"("distance"=w582, "Y"=-0.5, "X"=0.0, "RobotDriveDevRef"=w577) -> ("RobotDriveDevRef dup."=w573:T4)  [unwired: 7 in]
      n268 = String Subset(string=w575, offset (0)=1) -> (substring=w574:string)  [unwired: 1 in]
      n269 = case shown="\"R\", Default" w574 {
        tunnel: w573 -> [_ w585]
        frame "L" {
        }
        frame "R", Default {
          n270 = call "turn.vi"("Angle"=-90.0, "y"=-0.1, "RobotDriveDevRef"=w585) -> ()  [unwired: 8 in, 1 out]
        }
      }
    }
    frame "ultrasonic Test", Default {
      w586 = 0.0 ("X axis value")
      n271 = call <vilib>:"WPI_RobotDriveRefNum Registry Get.vi"("refnum name"="Drive") -> ("RobotDriveDevRef"=w588:T4)  [unwired: 9 in, 1 out]
      n272 = while {
        tunnel: w588 -> [w593]
        tunnel: [w595] -> _
        tunnel: [w592] -> w587
        stop <- w595 stop-if-true
        n273 = call-poly <vilib>:"WPI_UltrasonicRefNum Registry Get.vi"("refnum name"="Sonar") -> ("error out"=w599:errorcluster, "SonarSRF04DevRef"=w600:T11)  [unwired: 9 in]
        n274 = call-poly <vilib>:"WPI_UltrasonicGetRange.vi"("error in (no error)"=w599, "Range Units"=WPI_UltrasonicRangeUnits."inches", "SonarSRF04DevRef"=w600) -> ("Distance"=w597:dbl)  [unwired: 6 in, 2 out]
        n275 = call-poly <vilib>:"WPI_RobotDriveArcadeDrive.vi"("Y axis value"=-0.5 ("Y"), "X axis value"=0.0, "RobotDriveDevRef"=w593) -> ("RobotDriveDevRef"=w592:T4)  [unwired: 6 in, 2 out]
        n276 = Less?(x=w597, y=10.0 ("x")) -> (x < y?=w595:bool)
      }
      n277 = call-poly <vilib>:"WPI_RobotDriveArcadeDrive.vi"("Y axis value"=w586, "X axis value"=w586, "RobotDriveDevRef"=w587) -> ()  [unwired: 6 in, 3 out]
    }
  }
